vi "stop All Pumps.vi"(8 "error in (no error)":errorcluster) -> (0 "error out":errorcluster, 3 "function return":i32)   [LabVIEW 2018, in "AsiaPumpInterface.lvlib"]
doc: "extern ASIAPUMP_INTERFACE_API BOOL stopAllPumps();"
uses:
  <userlib>/AsiaPumpInterface/AsiaPumpInterface.lvlib
  <userlib>/AsiaPumpInterface/AsiaPumpInterface.dll
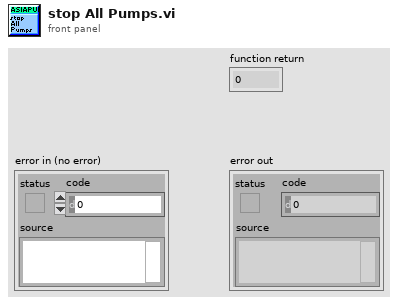
[diagram p1: front panel]
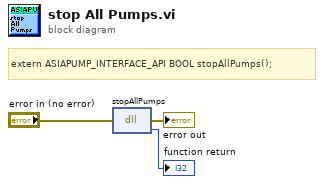
[diagram p0: block diagram]
diagram:
  # "extern ASIAPUMP_INTERFACE_API BOOL stopAllPumps();"
  n1 = dll-call lib="C:/Program Files (x86)/National Instruments/LabVIEW 2018/user.lib/AsiaPumpInterface/AsiaPumpInterface.*" fn="stopAllPumps"(error in="error in (no error)") -> (error out=→"error out":errorcluster, →"function return":i32)  [unwired: 2 in, 1 out]
